vi "FV_ME_MD.vi"(7 "do_reset":bool, 8 "error in":errorcluster, 10 "enable_or_disable":bool, 11 "VISA in":refnum<visa-resource-name>) -> (0 "error out":errorcluster, 1 "status":bool, 3 "VISA out":refnum<visa-resource-name>)   [LabVIEW 2019]
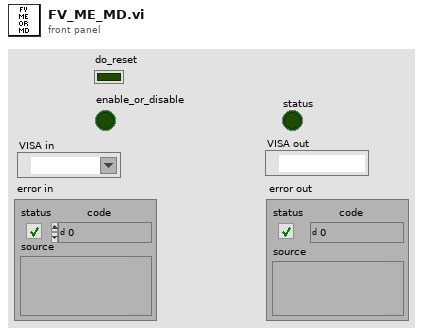
[diagram p1: front panel]
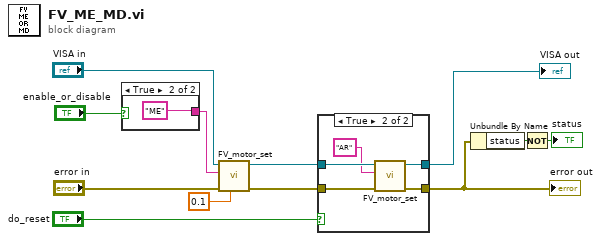
[diagram p0: block diagram]
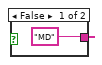
[diagram p3: hidden frame]
diagram:
  n1 = case shown="True" "enable_or_disable" {
    tunnel: ["MD" "ME"] -> w10
    frame False {
    }
    frame True {
    }
  }
  n2 = call "FV_motor_set.vi"("delay  (sec)"=0.1, "error in"="error in", "command"=w10, "VISA in"="VISA in") -> ("error out"=w5:errorcluster, "VISA out"=w4:refnum<visa-resource-name>)  [unwired: 6 in]
  n3 = case shown="True" "do_reset" {
    tunnel: w4 -> [w16 w21]
    tunnel: w5 -> [w15 w20]
    tunnel: [w15 w19] -> w3
    tunnel: [w16 w18] -> w2
    frame False {
    }
    frame True {
      n4 = call "FV_motor_set.vi"("error in"=w20, "command"="AR", "VISA in"=w21) -> ("error out"=w19:errorcluster, "VISA out"=w18:refnum<visa-resource-name>)  [unwired: 7 in]
    }
  }
  "error out" <- w3
  "VISA out" <- w2
  n5 = Unbundle By Name(w3) -> ("status"=w8:bool)
  n6 = Not(x=w8) -> (.not. x?=→"status":bool)
